vi "CPP_Initialise_puffer.vi"() -> (5 "Plug in titles":string[](array[string]), 7 "Plug in values":string[](array[string]))   [LabVIEW 2010]
uses:
  Controls/Post_Process.ctl
  ADAM Client/Sub VIs/ADAM Controls/Update_scan_value.ctl
  Globals/Meas_global.vi
  Globals/Extra_Commands_Global.vi
  Globals/Trav_pos_global.vi
  Globals/Preference_global.vi
  Globals/Dynamic_call_global.ph.vi
  Globals/Constants_global.vi
panel:
  out "DrainTime(s)":dbl format="%.2f"
  out "Case Currently On":string
  out "FillTime(s)":dbl format="%.2f"
  # "Fill and drain time are read from the ExtraCommand field, eg:\n!Puff Release=20;60"
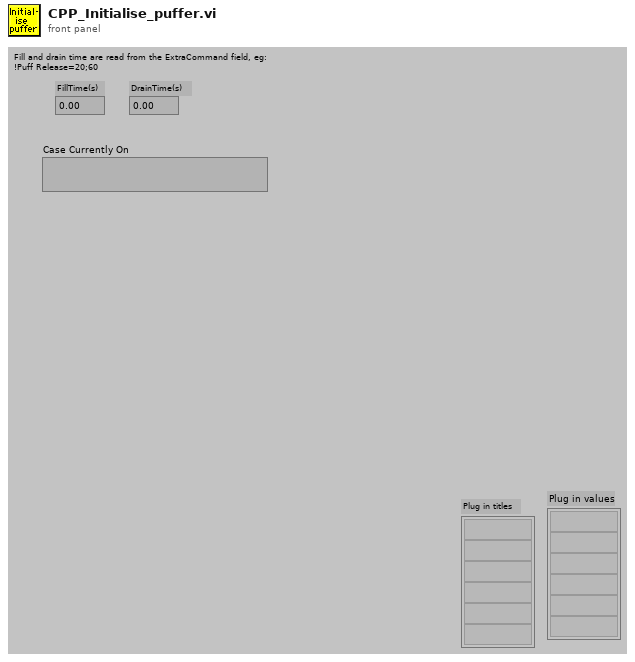
[diagram p1: front panel]
types:
  T1 = typedef "Post_Process.ctl" = enum16{"Take New Data", "Post Process Raw Data File"}
  T2 = typedef "Traverse_cluster.ctl" = cluster{"Start X":dbl, "Start Y":dbl, "Start Z":dbl, "End X":dbl, "End Y":dbl, "End Z":dbl, "No. of pts.":i32, "Spacing":T3, "Filename":path, "Tunnel Speed":dbl, "Averaging time (min)":dbl, "Extra Commands":string, "Specific Arguments":string, "Emission Rate (l/min)":dbl, "Trace Gas Concentration (%)":dbl, "Density Ratio":string, "Comments":string, "Row No":i32, "Row Type Selector":T4, "Completion time":string, "Row Duration (mins)":dbl, "No. of Valid pts.":i32, "Meas Setup File":string}
  T3 = typedef "Spacing.ctl" = enum16{"Linear", "Log", "Gauss", "Specified", "N/A"}
  T4 = typedef "Multi_run_mode.ctl" = enum16{"Move Traverse Only", "Set Tunnel Speed Only", "Set Source Only", "Set Measurement Conditions", "Single Measurement", "Vertical Profile", "Lateral Profile", "Longitudinal Profile", "Explore Volume", "Multi-Axis Profile", "Auto Calibrate", "Meas Fast FID Bkgnd", "Check Beam Power", "Scanning Valve Measurement", "Run VI Named:", "Set ADAM Ch", "Wait (minutes)", "Send Message", "Synchronize With:", "Fall Back to this Row", "Turn Off Row Repeating", "Blank Row"}
  T5 = typedef "Update_scan_value.ctl" = cluster{"Channel Name":string, "New Value":dbl}
  T6 = typedef "Rendezvous RefNum" = refnum<k1>
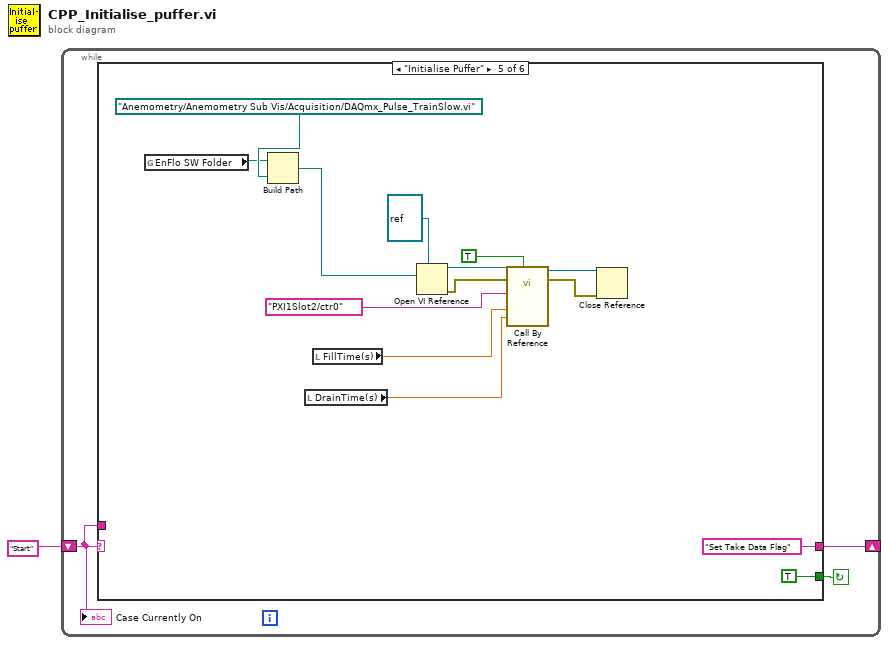
[diagram p0: block diagram]
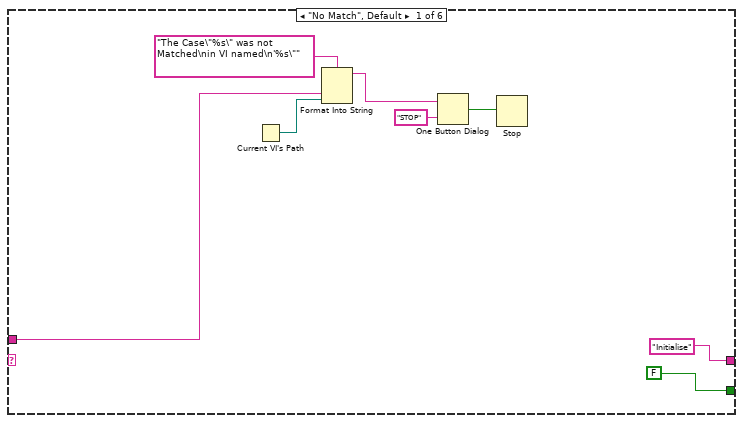
[diagram p2: hidden frame]
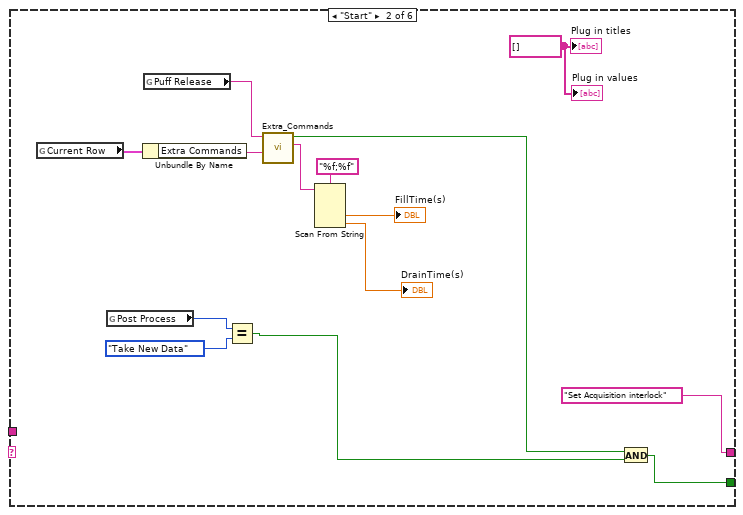
[diagram p3: hidden frame]
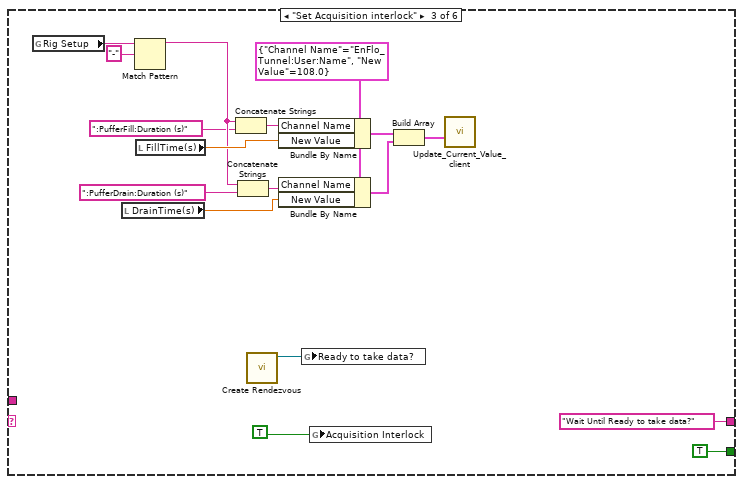
[diagram p4: hidden frame]
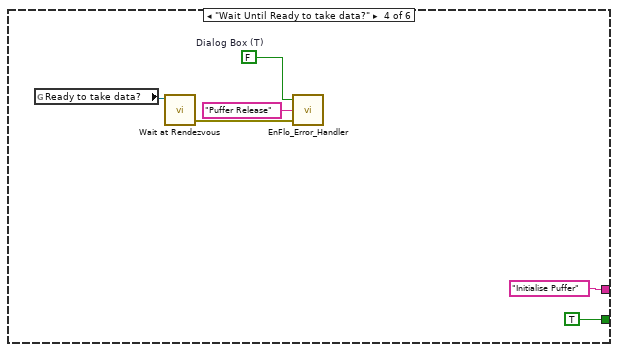
[diagram p5: hidden frame]
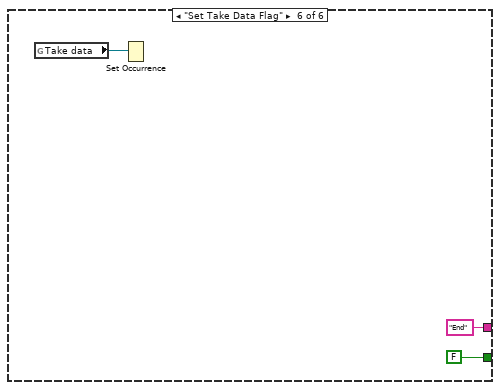
[diagram p6: hidden frame]
diagram:
  n1 = while {
    shift-left: "Start" -> [w2]
    shift-right: [w3] -> _
    stop <- w4 continue-if-true
    n2 = case shown="\"Initialise Puffer\"" w2 {
      tunnel: [FALSE w18 TRUE ("Command Found") TRUE ("Command Found") TRUE ("Command Found") FALSE ("Command Found")] -> w4
      tunnel: ["Initialise" "Set Acquisition interlock" "Wait Until Ready to take data?" "Initialise Puffer" "Set Take Data Flag" "End"] -> w3
      tunnel: w2 -> [w7 _ _ _ _ _]
      frame "No Match", Default {
        n3 = Current VI's Path() -> (path=w6:path)
        n4 = Format Into String(format string="The Case\"%s\" was not Matched\nin VI named\n'%s\"" ("Format String"), w7, w6) -> (resulting string=w10:string)  [unwired: 2 in, 1 out]
        n5 = One Button Dialog(message=w10, button name ("OK")="STOP") -> (true=w8:bool)
        n6 = Stop(stop? (T)=w8) -> ()
      }
      frame "Start" {
        w17 = string[] [] ("Plug in titles")
        n7 = global read "Trav_pos_global.vi" "Current Row"() -> (w26:T2)
        n8 = global read "Meas_global.vi" "Post Process"() -> (w21:T1)
        n9 = Unbundle By Name(w26) -> ("Extra Commands"=w24:string)
        n10 = global read "Extra_Commands_Global.vi" "Puff Release"() -> (w25:string)
        n11 = Equal?(x=w21, y=Post_Process."Take New Data" ("Post Process")) -> (x = y?=w19:bool)
        n12 = call "Extra_Commands.vi"("String to Search"=w24, "Command"=w25) -> ("String Value"=w16:string, "Command Found"=w20:bool)  [unwired: 2 in, 2 out]
        n13 = Scan From String(format string="%f;%f", input string=w16) -> (output 1=→"FillTime(s)":dbl, output 2=→"DrainTime(s)":dbl)  [unwired: 4 in, 3 out]
        n14 = And(x=w20, y=w19) -> (x .and. y?=w18:bool)
        "Plug in values" <- w17
        "Plug in titles" <- w17
      }
      frame "Set Acquisition interlock" {
        w35 = T5 {"Channel Name"="EnFlo_Tunnel:User:Name", "New Value"=108.0} ("Update Scan Value Cluster")
        n15 = global read "Preference_global.vi" "Rig Setup"() -> (w32:string)
        n16 = local read "DrainTime(s)"() -> (w34:dbl)
        n17 = Match Pattern(string=w32, regular expression="-") -> (before substring=w30:string)  [unwired: 4 out]
        n18 = local read "FillTime(s)"() -> (w38:dbl)
        n19 = Concatenate Strings(w30, ":PufferFill:Duration (s)") -> (w27:string)
        n20 = Concatenate Strings(w30, ":PufferDrain:Duration (s)") -> (w31:string)
        n21 = call <vilib>:"Create Rendezvous.vi"() -> ("rendezvous"=w40:T6)  [unwired: 5 in, 2 out]
        n22 = Bundle By Name(cluster=w35, "Channel Name"=w27, "New Value"=w38) -> (w37:T5)
        n23 = Bundle By Name(cluster=w35, "Channel Name"=w31, "New Value"=w34) -> (w36:T5)
        n24 = global write "Dynamic_call_global.ph.vi" "Ready to take data?"(w40) -> ()
        n25 = global write "Dynamic_call_global.ph.vi" "Acquisition Interlock"(TRUE ("Remote control")) -> ()
        n26 = Build Array(w37, w36) -> (w39:T5[])
        n27 = call "Update_Current_Value_client.vi"("Update array in"=w39) -> ()  [unwired: 1 in]
      }
      frame "Wait Until Ready to take data?" {
        w45 = FALSE  # Dialog Box (T)
        n28 = global read "Dynamic_call_global.ph.vi" "Ready to take data?"() -> (w48:T6)
        n29 = call <vilib>:"Wait at Rendezvous.vi"("rendezvous"=w48) -> ("error out"=w46:errorcluster)  [unwired: 4 in, 2 out]
        n30 = call "EnFlo_Error_Handler.vi"("error in (no error)"=w46, "Error Type"="Puffer Release", "Dialog Box (T)"=w45) -> ()  [unwired: 3 out]
      }
      frame "Initialise Puffer" {
        n31 = global read "Constants_global.vi" "EnFlo SW Folder"() -> (w54:path)
        n32 = Build Path(base path=w54, name or relative path=path "Anemometry/Anemometry Sub Vis/Acquisition/DAQmx_Pulse_TrainSlow.vi") -> (appended path=w56:path)
        n33 = local read "DrainTime(s)"() -> (w52:dbl)
        n34 = local read "FillTime(s)"() -> (w53:dbl)
        n35 = Open VI Reference(type specifier VI Refnum (for type only)=refnum<vi> refnum, vi path=w56) -> (vi reference=w57:refnum<vi>, error out=w60:errorcluster)  [unwired: 4 in]
        n36 = call-by-ref "?"(reference=w57, error in=w60, "Counter(s)"=tag "PXI1Slot2/ctr0", "Start?"=TRUE, "HighTime"=w53, "LowTime"=w52) -> (reference out=w59:refnum<vi>, error out=w61:errorcluster)  [unwired: 5 in]
        n37 = Close Reference(reference=w59, error in (no error)=w61) -> ()  [unwired: 1 out]
      }
      frame "Set Take Data Flag" {
        n38 = global read "Dynamic_call_global.ph.vi" "Take data"() -> (w64:refnum<k4>)
        n39 = Set Occurrence(w64) -> ()
      }
    }
    "Case Currently On" <- w2
  }
